vi "FPGA - Sampling Turbine.vi"() -> ()   [LabVIEW 2012]
uses:
  <vilib>/LabVIEW Targets/FPGA/cRIO/shared/nicrio_ModuleControls/nicrio_cRIO-9234_DataRatesRing2.ctl
  <vilib>/rvi/eio/common/nirviEmuTemplatePropertySet_noerrors.vi
  <vilib>/rvi/eio/common/nirviEmuTemplateMethod_errors.vi
  <vilib>/rvi/interface/RandomDataEmulation/nirviRandomDataFPGAFIFO.vi
  <vilib>/rvi/interface/RandomDataEmulation/niFpgaRandomDataHandleErrors.vi
  <vilib>/eio/EIOPropertyNode/EIOPropertyNode.xnode
  <vilib>/eio/EIONode/EIONode.xnode
  <vilib>/rvi/DataTransferAndStorage/Container/XNode/niFpgaContainer.xnode
  <vilib>/rvi/interface/RandomDataEmulation/nirviRandomDataFpgaReadWriteTemplate.vi
  <vilib>/rvi/eio/common/nirviEmuTemplatePropertyGet_errors.vi
  <vilib>/rvi/eio/common/nirviEmuTemplatePropertyGet_noerrors.vi
  <vilib>/rvi/eio/common/nirviEmuTemplatePropertySet_errors.vi
panel:
  in  "Turbine Max Voltage":fxp<+/-,20,5> format="%.17g"
  in  "Turbine PWM Period":fxp<+,32,32> caption="Turbine Period (mS)"
  in  "Turbine PWM Duty Cycle":fxp<+,32,0> caption="Turbine Duty Cycle"
  in  "Test Samples":u32
  in  "Down Sample Divisor":i32
  in  "Start Test?":bool
  out "Tach":fxp<+/-,24,4> format="%.22g"
  out "Tach Period (uSec/pulse)":u32
  in  "Data Rate":T1=1 items=["51.200 kS/s (NI 9234)"=1, "25.600 kS/s (NI 9234)"=2, "17.067 kS/s (NI 9234)"=3, "12.800 kS/s (NI 9234)"=4, "10.240 kS/s (NI 9234)"=5, "8.533 kS/s (NI 9234)"=6, "7.314 kS/s (NI 9234)"=7, "6.400 kS/s (NI 9234)"=8, "5.689 kS/s (NI 9234)"=9, "5.120 kS/s (NI 9234)"=10, "4.654 kS/s (NI 9234)"=11, "4.267 kS/s (NI 9234)"=12, "3.938 kS/s (NI 9234)"=13, "3.657 kS/s (NI 9234)"=14, "3.413 kS/s (NI 9234)"=15, "3.200 kS/s (NI 9234)"=16, "3.012 kS/s (NI 9234)"=17, "2.845 kS/s (NI 9234)"=18, "2.695 kS/s (NI 9234)"=19, "2.560 kS/s (NI 9234)"=20, "2.438 kS/s (NI 9234)"=21, "2.328 kS/s (NI 9234)"=22, "2.226 kS/s (NI 9234)"=23, "2.133 kS/s (NI 9234)"=24, "2.048 kS/s (NI 9234)"=25, "1.969 kS/s (NI 9234)"=26, "1.896 kS/s (NI 9234)"=27, "1.829 kS/s (NI 9234)"=28, "1.765 kS/s (NI 9234)"=29, "1.707 kS/s (NI 9234)"=30, "1.652 kS/s (NI 9234)"=31]
  out "Overflow Occurred":bool
  # "This FPGA VI acquires the\nacceleromter and tach\ndata from the NI 9234 and\nsupplies a control voltage for\nthe turbine speed through the\nNI 9263."
  # "NOTE: The front panel controls\nand indicators are for communication\nand debugging purposes only. Once\nthe FPGA VI is compiled it does not\nprovide a front panel."
  # "Inputs"
  # "Outputs"
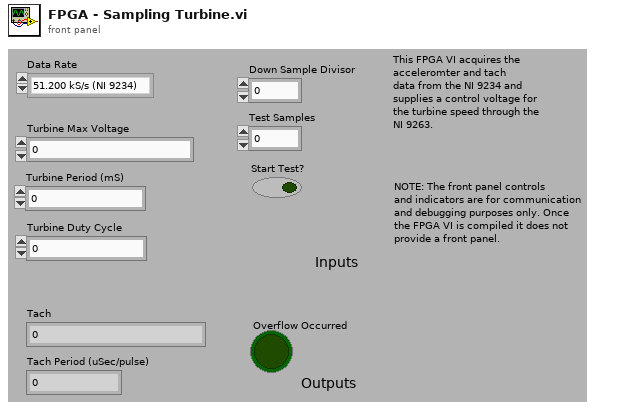
[diagram p1: front panel]
types:
  T1 = typedef "nicrio_cRIO-9234_DataRatesRing2.ctl" = u8
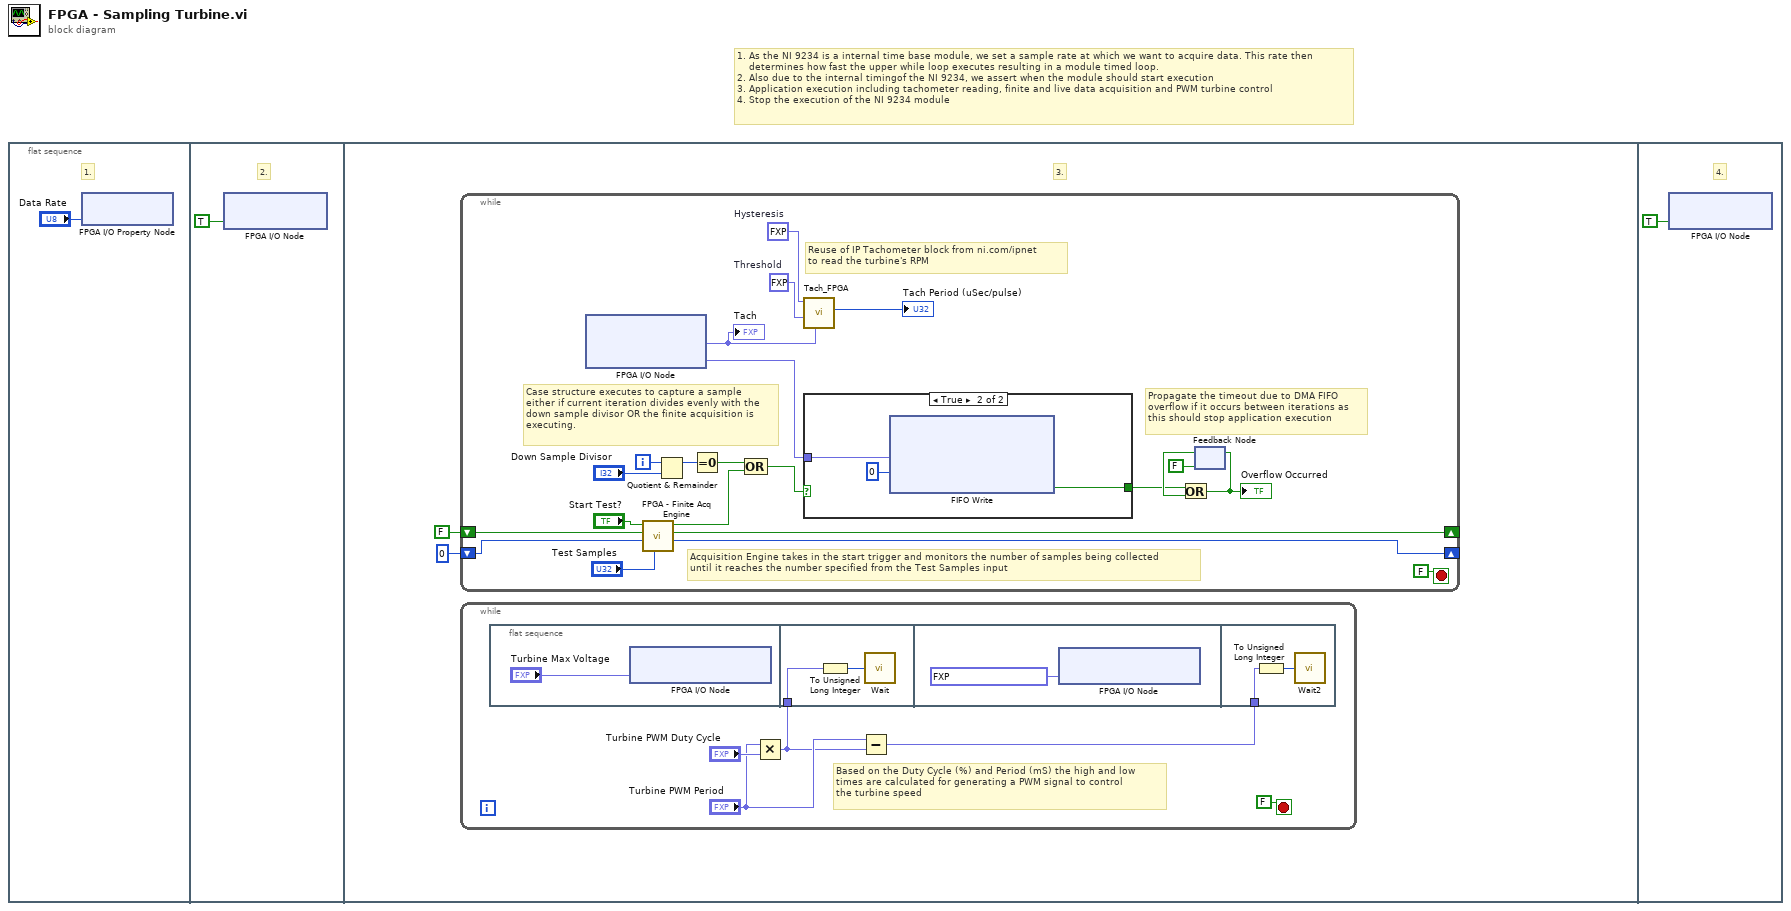
[diagram p0: block diagram]
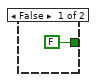
[diagram p2: hidden frame]
diagram:
  # "1. As the NI 9234 is a internal time base module, we set a sample rate at which we want to acquire data. This rate then\n    determines how fast the upper while loop executes resulting in a module timed loop. \n2. Also due to the internal timingof the NI 9234, we assert when the module should start execution\n3. Application execution including tachometer reading, finite and live data acquisition and PWM turbine control\n4. Stop the execution of the NI 9234 module"
  n1 = flat-sequence {
    frame #0 {
      # "1."
      n2 = xnode "FPGA I/O Property Node"("Data Rate"="Data Rate") -> ()  [unwired: 1 in, 1 out]
    }
    frame #1 {
      # "2."
      n3 = xnode "FPGA I/O Node"("Mod5/Start"=TRUE ("Mod2/Start")) -> ()  [unwired: 1 in, 1 out]
    }
    frame #2 {
      # "3."
      n4 = while {
        shift-right: [w19] -> _
        shift-left: u32 0 -> [w30]
        shift-right: [w24] -> _
        shift-left: FALSE -> [w28]
        i -> [w34]
        stop <- FALSE stop-if-true
        w36 = fxp<+/-,16,16> 2.0  # Threshold
        w17 = fxp<+,1,0> 0.5  # Hysteresis
        # "Propagate the timeout due to DMA FIFO\noverflow if it occurs between iterations as\nthis should stop application execution"
        # "Acquisition Engine takes in the start trigger and monitors the number of samples being collected\nuntil it reaches the number specified from the Test Samples input"
        # "Case structure executes to capture a sample\neither if current iteration divides evenly with the\ndown sample divisor OR the finite acquisition is\nexecuting."
        # "Reuse of IP Tachometer block from ni.com/ipnet\nto read the turbine's RPM"
        n5 = xnode "FPGA I/O Node"() -> ("Tach"=w16:fxp<+/-,24,4>, "Accelerometer"=w33:fxp<+/-,24,4>)  [unwired: 2 in, 2 out]
        "Tach" <- w16
        n6 = call "FPGA - Finite Acq Engine.vi"("Test Samples"="Test Samples", "Last Iteraction Samples Acq"=w30, "Continue Test?"=w28, "Start Test?"="Start Test?") -> ("Samples Acq"=w19:u32, "Continue Test"=w24:bool, "Sample?"=w27:bool)  [unwired: 5 in]
        n7 = Quotient & Remainder(x=w34, y="Down Sample Divisor") -> (x-y*floor(x/y)=w31:i32)  [unwired: 1 out]
        n8 = Equal To 0?(x=w31) -> (x = 0?=w26:bool)
        n9 = Compound Arithmetic op=OR(w26, w27) -> (w25:bool)
        n10 = call "Tach_FPGA.vi"("Analog In (Tach)"=w16, "Threshold"=w36, "Hysteresis"=w17) -> ("Tach Period (uSec/pulse)"=→"Tach Period (uSec/pulse)":u32)  [unwired: 7 in, 1 out]
        n11 = case shown="True" w25 {
          tunnel: [FALSE ("Timed Out?") w41] -> w21
          tunnel: w33 -> [_ w39]
          frame False {
          }
          frame True {
            n12 = xnode "FIFO Write"("Element"=w39, "Timeout"=0) -> ("Timed Out?"=w41:bool)  [unwired: 1 in, 1 out]
          }
        }
        n13 = feedback #1(FALSE ("Timed Out?")) -> (w22:bool)
        n14 = Or(x=w21, y=w22) -> (x .or. y?=w20:bool)
        "Overflow Occurred" <- w20
        n15 = feedback-in #1(w20) -> ()
      }
      n16 = while {
        stop <- FALSE stop-if-true
        # "Based on the Duty Cycle (%) and Period (mS) the high and low\ntimes are calculated for generating a PWM signal to control\nthe turbine speed"
        n17 = flat-sequence {
          tunnel: w6 -> [w11]
          tunnel: w5 -> [w14]
          frame #0 {
            n18 = xnode "FPGA I/O Node"("Turbine Speed Ctrl"="Turbine Max Voltage") -> ()  [unwired: 1 in, 1 out]
          }
          frame #1 {
            n19 = To Unsigned Long Integer(number=w11) -> (unsigned 32bit integer=w12:u32)
            n20 = call "Wait"("Count(mSec)"=w12) -> ()  [unwired: 1 out]
          }
          frame #2 {
            n21 = xnode "FPGA I/O Node"("Turbine Speed Ctrl"=fxp<+/-,20,5> 0.0 ("Mod1/AO0")) -> ()  [unwired: 1 in, 1 out]
          }
          frame #3 {
            n22 = To Unsigned Long Integer(number=w14) -> (unsigned 32bit integer=w15:u32)
            n23 = call "Wait2"("Count(mSec)"=w15) -> ()  [unwired: 1 out]
          }
        }
        n24 = Multiply(x="Turbine PWM Period", y="Turbine PWM Duty Cycle") -> (x*y=w6:fxp<+,32,32>)
        n25 = Subtract(x="Turbine PWM Period", y=w6) -> (x-y=w5:fxp<+/-,32,32>)
      }
    }
    frame #3 {
      # "4."
      n26 = xnode "FPGA I/O Node"("Mod5/Stop"=TRUE ("Mod2/Stop")) -> ()  [unwired: 1 in, 1 out]
    }
  }
